vi "IsXBetween.vi"(1 "z":dbl, 2 "y":dbl, 3 "x":dbl) -> (0 "(y-z) < x < (y+z)":bool)   [LabVIEW 2019]
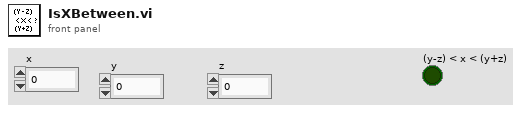
[diagram p1: front panel]
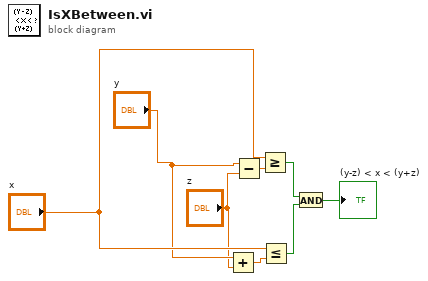
[diagram p0: block diagram]
diagram:
  n1 = Add(x="y", y="z") -> (x+y=w4:dbl)
  n2 = Subtract(x="y", y="z") -> (x-y=w1:dbl)
  n3 = Greater Or Equal?(x="x", y=w1) -> (x >= y?=w7:bool)
  n4 = Less Or Equal?(x="x", y=w4) -> (x <= y?=w8:bool)
  n5 = And(x=w7, y=w8) -> (x .and. y?=→"(y-z) < x < (y+z)":bool)
